vi "S30c_dll F48.vi"(4 "error in":errorcluster, 7 "Dev Addr":u8=250) -> (0 "error out":errorcluster, 1 "Info":T1, 2 "SW-Version":string)   [LabVIEW 2014, in "K_S30c_dll.lvlib"]
uses:
  K_S30c_dll.lvlib
  s30c.dll
panel:
  # "Function 48: ini \n\nusing s30c.dll\nKeller AG für Druckmesstechnik, 29.5.08 b.v."
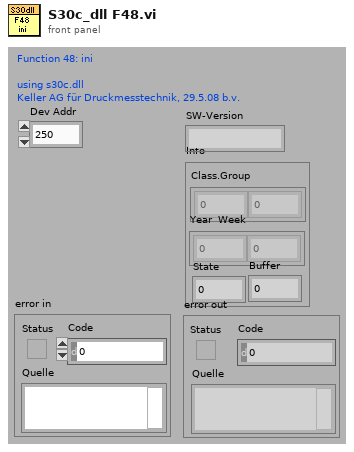
[diagram p1: front panel]
types:
  T1 = cluster{"Class.Group":u8[], "Year  Week":u8[], "State":u8, "Buffer":u8}
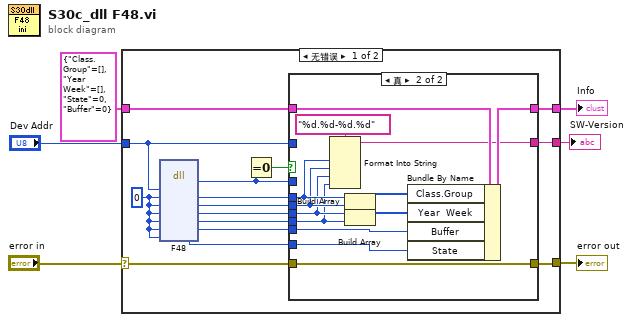
[diagram p0: block diagram]
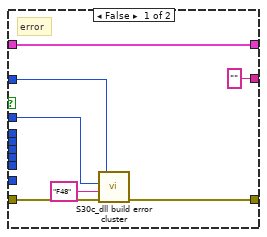
[diagram p2: hidden frame]
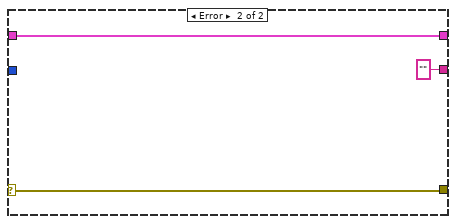
[diagram p3: hidden frame]
diagram:
  n1 = case shown="无错误" "error in" {
    selector: "error in" -> [w18 w44]
    tunnel: [w17 w44] -> w3
    tunnel: "Dev Addr" -> [w12 _]
    tunnel: [w19 w43] -> w5
    tunnel: T1 {"Class.Group"=[], "Year  Week"=[], "State"=0, "Buffer"=0} ("Info") -> [w16 w43]
    tunnel: [w7 ""] -> w2
    frame No Error {
      w21 = u8 0 ("Class")
      n2 = dll-call lib="PTH2Labs EworkSINOPEC北控自动相渗software2.08.5_dlls30c.dll" fn="F48"("DevAddr"=w12, "Class"=w21, "Group"=w21, "Year"=w21, "Week"=w21, "Buffer"=w21, "State"=w21) -> (w13:i16, "Class"=w11:u8, "Group"=w10:u8, "Year"=w9:u8, "Week"=w8:u8, "Buffer"=w15:u8, "State"=w14:u8)  [unwired: 4 in, 2 out]
      n3 = Equal To 0?(x=w13) -> (x = 0?=w20:bool)
      n4 = case shown="真" w20 {
        tunnel: w16 -> [w28 w41]
        tunnel: [w28 w40] -> w19
        tunnel: w18 -> [w27 w39]
        tunnel: [w26 w39] -> w17
        tunnel: w15 -> [_ w38]
        tunnel: w14 -> [_ w37]
        tunnel: w13 -> [w23 _]
        tunnel: w12 -> [w24 _]
        tunnel: w11 -> [_ w33]
        tunnel: w10 -> [_ w32]
        tunnel: w9 -> [_ w31]
        tunnel: w8 -> [_ w30]
        tunnel: ["" w29] -> w7
        frame False {
          # "error"
          n5 = call "S30c_dll build error cluster.vi"("error in"=w27, "error Text"="F48", "error code"=w23, "Dev Addr"=w24) -> ("error out"=w26:errorcluster)  [unwired: 3 in]
        }
        frame True {
          n6 = Format Into String(format string="%d.%d-%d.%d" ("Format-String"), w33, w32, w31, w30) -> (resulting string=w29:string)  [unwired: 2 in, 1 out]
          n7 = Build Array(w33, w32) -> (w35:u8[])
          n8 = Build Array(w31, w30) -> (w36:u8[])
          n9 = Bundle By Name(cluster=w41, "Class.Group"=w35, "Year  Week"=w36, "Buffer"=w38, "State"=w37) -> (w40:T1)
        }
      }
    }
    frame Error {
    }
  }
  "Info" <- w5
  "error out" <- w3
  "SW-Version" <- w2
